vi "ap get id and board version.vi"(9 "dest_board_version":u32, 10 "dest_id":u32, 11 "ap_handle":u32) -> (1 "dest_board_version out":u32, 2 "dest_id out":u32, 3 "ap_handle out":u32, 5 "function return":i32)   [LabVIEW 2019, in "apdm.lvlib"]
doc: "APDM_EXPORT int apdm_ap_get_id_and_board_version(apdm_ap_handle_t ap_handle, uint32_t *dest_id, uint32_t *dest_board_version);"
uses:
  apdm.lvlib
  Lee Lab/CP FES Walking 2018/Code/Working/LabVIEW/apdm.dll
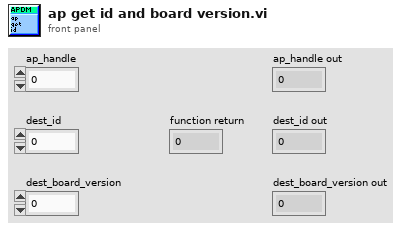
[diagram p1: front panel]
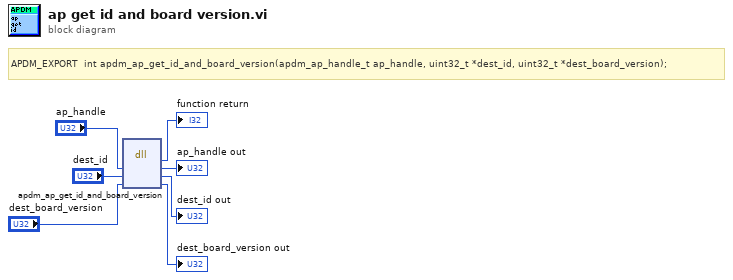
[diagram p0: block diagram]
diagram:
  # "APDM_EXPORT  int apdm_ap_get_id_and_board_version(apdm_ap_handle_t ap_handle, uint32_t *dest_id, uint32_t *dest_board_version);"
  n1 = dll-call lib="C:/Users/jfalesi/Dropbox/Lee Lab/CP FES Walking 2018/Code/Working/LabVIEW/apdm.*" fn="apdm_ap_get_id_and_board_version"("ap_handle"="ap_handle", "dest_id"="dest_id", "dest_board_version"="dest_board_version") -> (→"function return":i32, "ap_handle"=→"ap_handle out":u32, "dest_id"=→"dest_id out":u32, "dest_board_version"=→"dest_board_version out":u32)  [unwired: 3 in, 2 out]
